vi "From MsgPack bytes.vi"(8 "error in (no error)":errorcluster, 11 "bytes":u8[](array[numeric]) format="%x") -> (0 "error out":errorcluster, 2 "Message Type":T1, 3 "MsgPackMessage":refnum<class "WampMessage MsgPack.lvclass">)   [LabVIEW 2020, in "wamplv.lvlib" / "WampMessage MsgPack.lvclass"]
uses:
  WampMessage MsgPack.lvclass
  TypeDefs/WAMP Message Codes.ctl
  MessagePack/MessagePackNumeric/MessagePackNumeric.lvclass/MessagePackNumeric.ctl
  WampMessage MsgPack.lvclass/WampMessage MsgPack.ctl
  9d5ab1ec-4292-4d6f-8c29-874e9731c837.vi
  MessagePack/MessagePackNumeric/Direct cast/as INT8.vi
  MessagePack/MessagePackNumeric/Direct cast/as SGl.vi
  MessagePack/MessagePackNumeric/Direct cast/as DBL.vi
  MessagePack/MessagePackNumeric/Direct cast/as UINT8.vi
  MessagePack/MessagePackNumeric/Direct cast/as UINT16.vi
  MessagePack/MessagePackNumeric/Direct cast/as UINT32.vi
  MessagePack/MessagePackNumeric/Direct cast/as UINT64.vi
  MessagePack/MessagePackNumeric/Direct cast/as INT16.vi
  MessagePack/MessagePackNumeric/Direct cast/as INT32.vi
  MessagePack/MessagePackNumeric/Direct cast/as INT64.vi
  MessagePack/MessagePackNumeric/Accessors/Read Type.vi
  MessagePack/MessagePackNumeric/Accessors/Read Numeric Bytes.vi
  <vilib>/Utility/error.llb/Error Cluster From Error Code.vi
  MessagePack/MsgPackArray/MsgPackArray.lvclass
  MessagePack/MessagePackNumeric/MessagePackNumeric.lvclass
  wamplv.lvlib
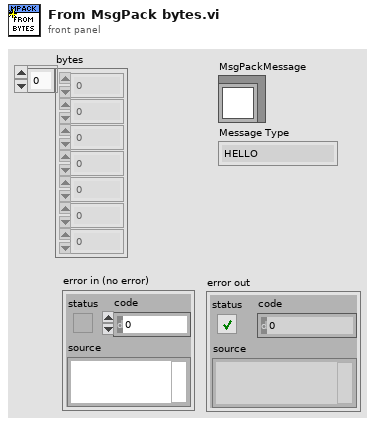
[diagram p1: front panel]
types:
  T1 = typedef "wamplv.lvlib/WAMP Message Codes.ctl" = enum8{"HELLO", "WELCOME", "CHALLENGE", "AUTHENTICATE", "ABORT", "GOODBYE", "ERROR", "PUBLISH", "PUBLISHED", "SUBSCRIBE", "SUBSCRIBED", "UNSUBSCRIBE", "UNSUBSCRIBED", "EVENT", "CALL", "RESULT", "REGISTER", "REGISTERED", "UNREGISTER", "UNREGISTERED", "INVOCATION", "YIELD"}
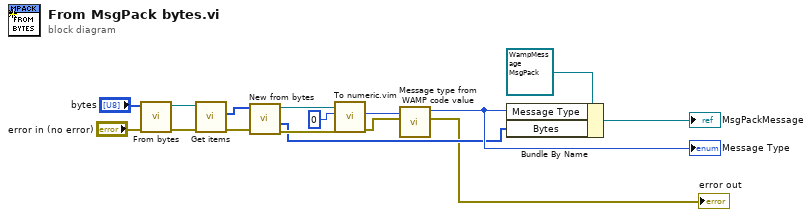
[diagram p0: block diagram]
diagram:
  n1 = call "From bytes.vi"("error in (no error)"="error in (no error)", "bytes"="bytes") -> ("error out"=w15:errorcluster, "MsgPackArray out"=w16:refnum<class "MsgPackArray.lvclass">)  [unwired: 8 in]
  n2 = call "Get items.vi"("error in (no error)"=w15, "MsgPackArray in"=w16) -> ("error out"=w14:errorcluster, "Bytes"=w13:u8[])  [unwired: 7 in, 1 out]
  n3 = call "New from bytes.vi"("error in (no error)"=w14, "Bytes"=w13) -> ("error out"=w11:errorcluster, "remaining bytes"=w3:u8[], "MessagePackNumeric out"=w12:refnum<class "MessagePackNumeric.lvclass">)  [unwired: 6 in, 1 out]
  n4 = call "To numeric.vim"("error in (no error)"=w11, "Numeric Type"=u8 0, "MessagePackNumeric in"=w12) -> ("error out"=w6:errorcluster, "Reult"=w7:u8)  [unwired: 6 in, 1 out]
  n5 = call "Message type from WAMP code value.vi"("error IO"=w6, "WAMP Numeric value"=w7) -> ("error out"=→"error out":errorcluster, "Message Type"=w4:T1)  [unwired: 6 in]
  "Message Type" <- w4
  n6 = Bundle By Name(cluster=refnum<class "WampMessage MsgPack.lvclass"> refnum ("wamplv.lvlib:MsgPackMessage.lvclass"), "Message Type"=w4, "Bytes"=w3) -> (→"MsgPackMessage":refnum<class "WampMessage MsgPack.lvclass">)
